vi "1_2.vi"() -> ()   [LabVIEW 2021]
panel:
  out "error out":errorcluster
  out "Answer to Submit":i32
  # "Advent Of Code 2021"
  # "Check block diagram for the code"
  # "patrik karandusovsky\npatrik.karandusovsky@gmail.com"
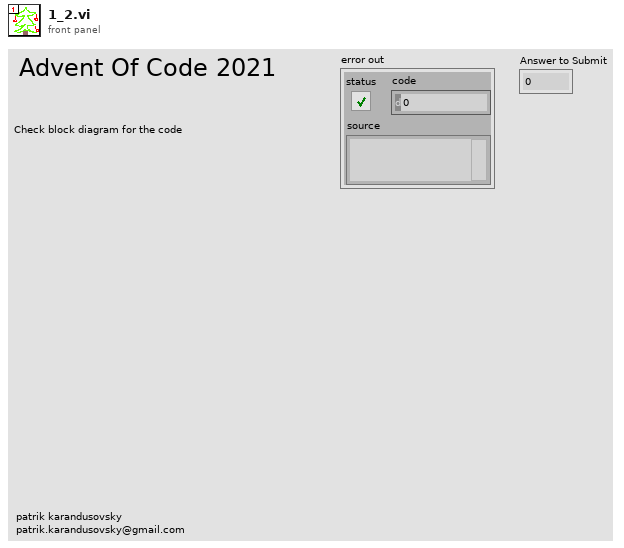
[diagram p1: front panel]
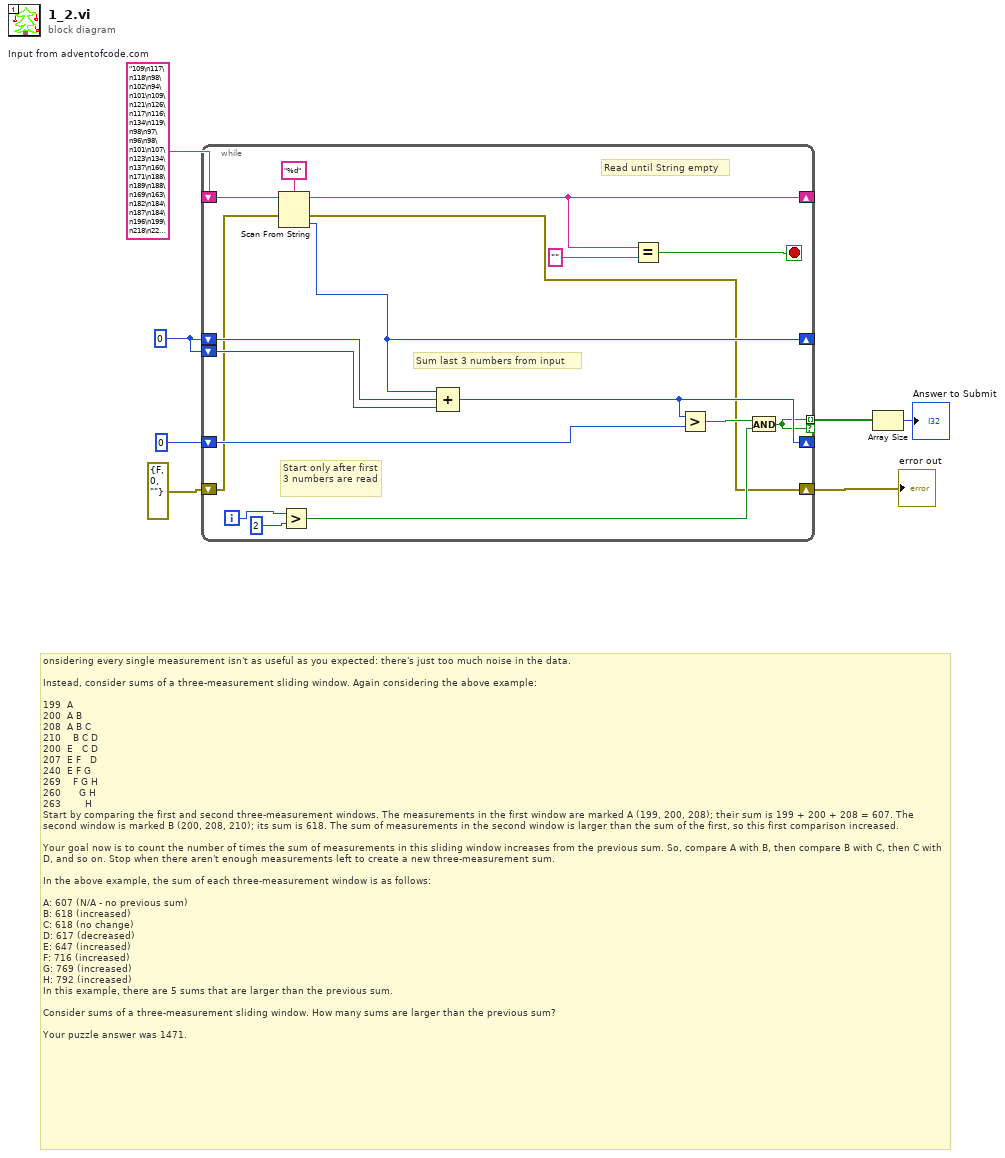
[diagram p0: block diagram]
diagram:
  w7 = "109\n117\n118\n98\n102\n94\n101\n109\n121\n126\n117\n116\n134\n119\n98\n97\n96\n98\n101\n107\n123\n134\n137\n160\n171\n188\n189\n188\n169\n163\n182\n184\n187\n184\n196\n199\n218\n222\n223\n218\n214\n220\n215\n223\n226\n228\n236\n237\n268\n277\n282\n284\n285\n288\n289\n313\n322\n331\n335\n331\n316\n323\n314\n313\n314\n301\n302\n320\n315\n323\n324\n346\n347\n362\n376\n377\n378\n379\n381\n391\n392\n395\n391\n393\n399\n401\n403\n428\n423\n422\n427\n430\n432\n431\n433\n449\n456\n455\n456\n457\n456\n460\n461\n460\n459\n460\n467\n468\n505\n506\n513\n505\n509\n510\n511\n521\n522\n523\n525\n521\n514\n517\n510\n507\n534\n543\n554\n552\n578\n587\n593\n598\n591\n592\n579\n580\n576\n594\n593\n594\n598\n610\n611\n609\n607\n606\n609\n616\n617\n605\n604\n61..."  # Input from adventofcode.com
  w4 = 0
  # "onsidering every single measurement isn't as useful as you expected: there's just too much noise in the data.\n\nInstead, consider sums of a three-measurement sliding window. Again considering the above example:\n\n199  A      \n200  A B    \n208  A B C  \n210    B C D\n200  E   C D\n207  E F   D\n240  E F G  \n269    F G H\n260      G H\n263        H\nStart by comparing the first and second three-measurement windows. The measurements in the first window are marked A (199, 200, 208); their sum is 199 + 200 + 208 = 607. The second window is marked B (200, 208, 210); its sum is 618. The sum of measurements in the second window is larger than the sum of the first, so this first comparison increased.\n\nYour goal now is to count the number of times the sum of measurements in this sliding window increases from the previous sum. So, compare A with B, then compare B with C, then C with D, and so on. Stop when there aren't enough measurements left to create a new three-measurement sum.\n\nIn the above example, the sum of each three-measurement window is as follows:\n\nA: 607 (N/A - no previous sum)\nB: 618 (increased)\nC: 618 (no change)\nD: 617 (decreased)\nE: 647 (increased)\nF: 716 (increased)\nG: 769 (increased)\nH: 792 (increased)\nIn this example, there are 5 sums that are larger than the previous sum.\n\nConsider sums of a three-measurement sliding window. How many sums are larger than the previous sum?\n\nYour puzzle answer was 1471."
  n1 = while {
    shift-right: [w22] -> _
    shift-left: w7 -> [w24]
    shift-right: [w15] -> _
    shift-left: w4 -> [w19]
    shift-right: [w17] -> _
    shift-left: 0 -> [w16]
    shift-left: w4 -> [w18]
    tunnel: [w11] -> w3 mode=indexing if=w11
    shift-right: [w8] -> w1
    shift-left: errorcluster {"status"=FALSE, "code"=0, "source"=""} ("error in (no error)") -> [w9]
    i -> [w14]
    stop <- w20 stop-if-true
    # "Start only after first 3 numbers are read"
    # "Sum last 3 numbers from input"
    # "Read until String empty"
    n2 = Scan From String(format string="%d", input string=w24, error in=w9) -> (remaining string=w22:string, error out=w8:errorcluster, output 1=w15:i32)  [unwired: 2 in, 1 out]
    n3 = Greater?(x=w14, y=2) -> (0:w10:bool)
    n4 = Compound Arithmetic op=ADD(w15, w19, w18) -> (w17:i32)
    n5 = Equal?(x=w22, y="") -> (x = y?=w20:bool)
    n6 = Greater?(x=w17, y=w16) -> (0:w12:bool)
    n7 = And(x=w12, y=w10) -> (x .and. y?=w11:bool)
  }
  "error out" <- w1
  n8 = Array Size(array=w3) -> (size(s)=→"Answer to Submit":i32)
